vi "validate.vi"(8 "error in":errorcluster, 11 "Add Module configuration in":refnum<class "Add Module configuration.lvclass">) -> (0 "error out":errorcluster, 3 "Add Module configuration out":refnum<class "Add Module configuration.lvclass">)   [LabVIEW 2018, in "Add Module configuration.lvclass"]
doc: "This function performs validation of the configuration. This function should be safe to call at any point and should not rely on anything in the runtime environment."
uses:
  Add Module configuration.lvclass
  <vilib>/NI/Tag Bus Module Framework/module configuration/TBM module configuration.lvclass
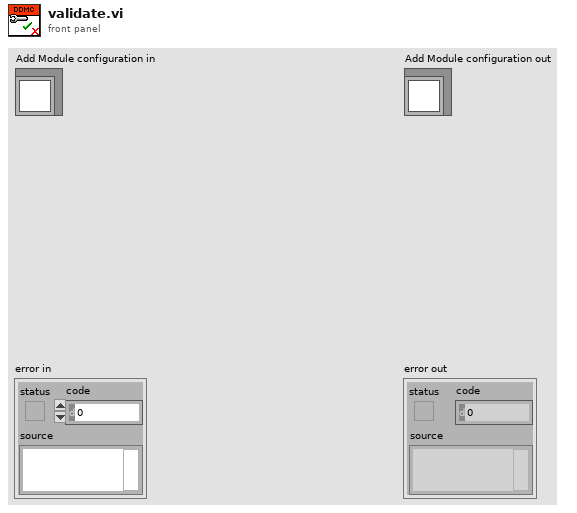
[diagram p1: front panel]
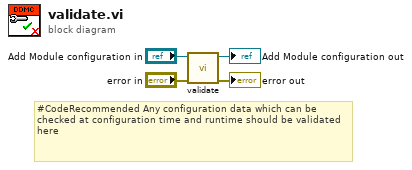
[diagram p0: block diagram]
diagram:
  # "#CodeRecommended Any configuration data which can be checked at configuration time and runtime should be validated here"
  n1 = call-parent "validate.vi"("error in"="error in", "configuration in"="Add Module configuration in") -> ("error out"=→"error out":errorcluster, "configuration out"=→"Add Module configuration out":refnum<class "Add Module configuration.lvclass">)  [unwired: 8 in]
